vi "UsrProfiles-Parse param names.vi"(10 "key":string, 11 "Saved value":dbl) -> (3 "String":string)   [LabVIEW 2020]
uses:
  Typedefs/Movement mode.ctl
  Typedefs/Reference source.ctl
  Movement Correction/Typedefs/Control algorithm.ctl
  Typedefs/Channel Selector.ctl
  Typedefs/Line draw mode.ctl
  Typedefs/Imaging Protocols enum.ctl
  Typedefs/AOL modes.ctl
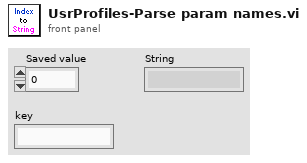
[diagram p1: front panel]
types:
  T1 = typedef "Movement mode.ctl" = enum16{"Move the frame", "Move the feature"}
  T2 = typedef "Reference source.ctl" = enum16{"Green channel", "Red channel"}
  T3 = typedef "Control algorithm.ctl" = enum16{"PID", "Kalman"}
  T4 = typedef "Channel Selector.ctl" = enum16{"Red Channel", "Green Channel", "Blended"}
  T5 = enum16{"Grayscale", "Binary", "Gradient", "Rainbow", "Temperature", "User Defined"}
  T6 = typedef "Line draw mode.ctl" = enum16{"Free draw", "Orthogonal"}
  T7 = typedef "Imaging Protocols enum.ctl" = enum16{"AOL Z-Stack", "Motor Z Stack", "Functional Acquisition", "Single Plane Acquisition", "Volume Acquisition", "Live Imaging", "Live Plane Imaging", "Live Volume Imaging"}
  T8 = typedef "AOL modes.ctl" = enum16{"Raster", "Structural", "Pointing", "Mini Scan", "Alignment"}
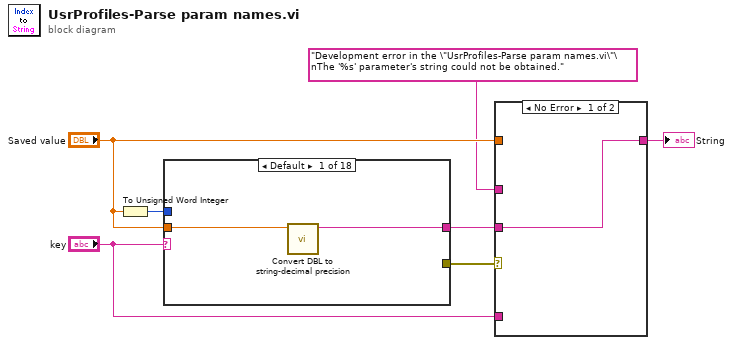
[diagram p0: block diagram]
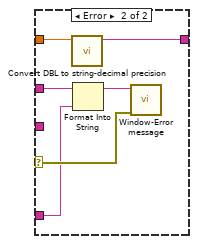
[diagram p2: hidden frame]
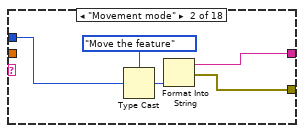
[diagram p3: hidden frame]
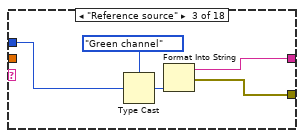
[diagram p4: hidden frame]
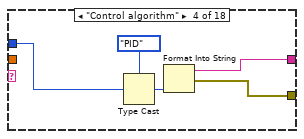
[diagram p5: hidden frame]
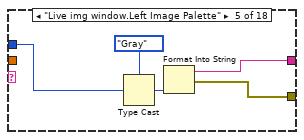
[diagram p6: hidden frame]
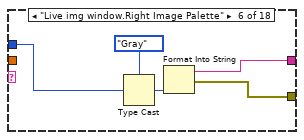
[diagram p7: hidden frame]
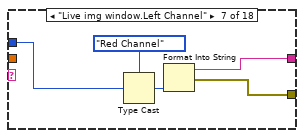
[diagram p8: hidden frame]
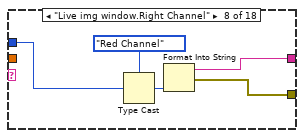
[diagram p9: hidden frame]
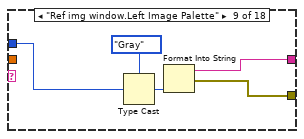
[diagram p10: hidden frame]
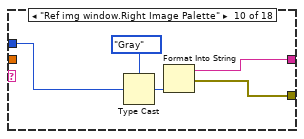
[diagram p11: hidden frame]
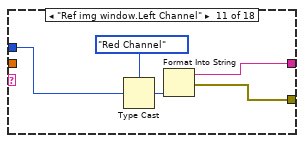
[diagram p12: hidden frame]
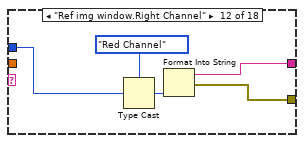
[diagram p13: hidden frame]
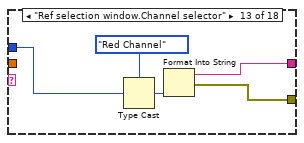
[diagram p14: hidden frame]
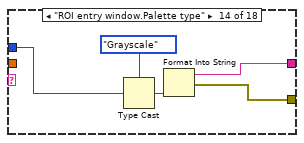
[diagram p15: hidden frame]
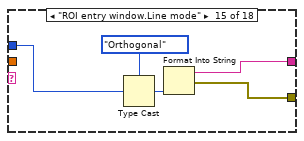
[diagram p16: hidden frame]
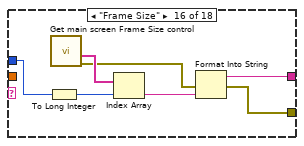
[diagram p17: hidden frame]
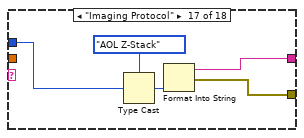
[diagram p18: hidden frame]
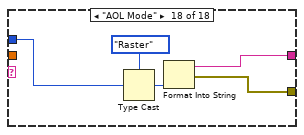
[diagram p19: hidden frame]
diagram:
  n1 = To Unsigned Word Integer(number="Saved value") -> (unsigned 16bit integer=w7:u16)
  n2 = case shown="Default" "key" {
    tunnel: w7 -> [_ w14 w19 w24 w29 w34 w39 w44 w49 w54 w59 w64 w69 w74 w79 w84 w91 w96]
    tunnel: [w8 w11 w17 w22 w27 w32 w37 w42 w47 w52 w57 w62 w67 w72 w77 w86 w89 w94] -> w4
    tunnel: [_ w10 w15 w20 w26 w31 w36 w41 w46 w51 w56 w61 w66 w71 w76 w85 w88 w93] -> w6
    tunnel: "Saved value" -> [w9 _ _ _ _ _ _ _ _ _ _ _ _ _ _ _ _ _]
    frame Default {
      n3 = call <userlib>:"Convert DBL to string-decimal precision.vi"("DBL Value"=w9) -> ("Converted to String"=w8:string)  [unwired: 10 in]
    }
    frame "Movement mode" {
      n4 = Type Cast(type=Movement_mode."Move the feature" ("Movement mode"), x=w14) -> (*(type *) &x=w13:T1)
      n5 = Format Into String(w13) -> (resulting string=w11:string, error out=w10:errorcluster)  [unwired: 3 in]
    }
    frame "Reference source" {
      n6 = Type Cast(type=Reference_source."Green channel" ("Reference Source"), x=w19) -> (*(type *) &x=w18:T2)
      n7 = Format Into String(w18) -> (resulting string=w17:string, error out=w15:errorcluster)  [unwired: 3 in]
    }
    frame "Control algorithm" {
      n8 = Type Cast(type=Control_algorithm."PID" ("Control algorithm"), x=w24) -> (*(type *) &x=w23:T3)
      n9 = Format Into String(w23) -> (resulting string=w22:string, error out=w20:errorcluster)  [unwired: 3 in]
    }
    frame "Live img window.Left Image Palette" {
      n10 = Type Cast(type=enum16{"Gray", "Red", "Green"}."Gray" ("Value"), x=w29) -> (*(type *) &x=w28:enum16{"Gray", "Red", "Green"})
      n11 = Format Into String(w28) -> (resulting string=w27:string, error out=w26:errorcluster)  [unwired: 3 in]
    }
    frame "Live img window.Right Image Palette" {
      n12 = Type Cast(type=enum16{"Gray", "Red", "Green"}."Gray" ("Value"), x=w34) -> (*(type *) &x=w33:enum16{"Gray", "Red", "Green"})
      n13 = Format Into String(w33) -> (resulting string=w32:string, error out=w31:errorcluster)  [unwired: 3 in]
    }
    frame "Live img window.Left Channel" {
      n14 = Type Cast(type=Channel_Selector."Red Channel" ("Value"), x=w39) -> (*(type *) &x=w38:T4)
      n15 = Format Into String(w38) -> (resulting string=w37:string, error out=w36:errorcluster)  [unwired: 3 in]
    }
    frame "Live img window.Right Channel" {
      n16 = Type Cast(type=Channel_Selector."Red Channel" ("Value"), x=w44) -> (*(type *) &x=w43:T4)
      n17 = Format Into String(w43) -> (resulting string=w42:string, error out=w41:errorcluster)  [unwired: 3 in]
    }
    frame "Ref img window.Left Image Palette" {
      n18 = Type Cast(type=enum16{"Gray", "Red", "Green"}."Gray" ("Value"), x=w49) -> (*(type *) &x=w48:enum16{"Gray", "Red", "Green"})
      n19 = Format Into String(w48) -> (resulting string=w47:string, error out=w46:errorcluster)  [unwired: 3 in]
    }
    frame "Ref img window.Right Image Palette" {
      n20 = Type Cast(type=enum16{"Gray", "Red", "Green"}."Gray" ("Value"), x=w54) -> (*(type *) &x=w53:enum16{"Gray", "Red", "Green"})
      n21 = Format Into String(w53) -> (resulting string=w52:string, error out=w51:errorcluster)  [unwired: 3 in]
    }
    frame "Ref img window.Left Channel" {
      n22 = Type Cast(type=Channel_Selector."Red Channel" ("Value"), x=w59) -> (*(type *) &x=w58:T4)
      n23 = Format Into String(w58) -> (resulting string=w57:string, error out=w56:errorcluster)  [unwired: 3 in]
    }
    frame "Ref img window.Right Channel" {
      n24 = Type Cast(type=Channel_Selector."Red Channel" ("Value"), x=w64) -> (*(type *) &x=w63:T4)
      n25 = Format Into String(w63) -> (resulting string=w62:string, error out=w61:errorcluster)  [unwired: 3 in]
    }
    frame "Ref selection window.Channel selector" {
      n26 = Type Cast(type=Channel_Selector."Red Channel" ("Value"), x=w69) -> (*(type *) &x=w68:T4)
      n27 = Format Into String(w68) -> (resulting string=w67:string, error out=w66:errorcluster)  [unwired: 3 in]
    }
    frame "ROI entry window.Palette type" {
      n28 = Type Cast(type=T5."Grayscale" ("Value"), x=w74) -> (*(type *) &x=w73:T5)
      n29 = Format Into String(w73) -> (resulting string=w72:string, error out=w71:errorcluster)  [unwired: 3 in]
    }
    frame "ROI entry window.Line mode" {
      n30 = Type Cast(type=Line_draw_mode."Orthogonal" ("Value"), x=w79) -> (*(type *) &x=w78:T6)
      n31 = Format Into String(w78) -> (resulting string=w77:string, error out=w76:errorcluster)  [unwired: 3 in]
    }
    frame "Frame Size" {
      n32 = To Long Integer(number=w84) -> (32bit integer=w83:i32)
      n33 = call "Get main screen Frame Size control.vi"() -> ("error out"=w80:errorcluster, "Strings []"=w81:string[])  [unwired: 9 in, 1 out]
      n34 = Index Array(array=w81, index=w83) -> (element=w82:string)
      n35 = Format Into String(error in=w80, w82) -> (resulting string=w86:string, error out=w85:errorcluster)  [unwired: 2 in]
    }
    frame "Imaging Protocol" {
      n36 = Type Cast(type=Imaging_Protocols_enum."AOL Z-Stack" ("Imaging Protocol"), x=w91) -> (*(type *) &x=w90:T7)
      n37 = Format Into String(w90) -> (resulting string=w89:string, error out=w88:errorcluster)  [unwired: 3 in]
    }
    frame "AOL Mode" {
      n38 = Type Cast(type=AOL_modes."Raster" ("AOL Mode"), x=w96) -> (*(type *) &x=w95:T8)
      n39 = Format Into String(w95) -> (resulting string=w94:string, error out=w93:errorcluster)  [unwired: 3 in]
    }
  }
  n40 = case shown="No Error" w6 {
    selector: w6 -> [_ w99]
    tunnel: "Saved value" -> [_ w103]
    tunnel: w4 -> [w97 _]
    tunnel: [w97 w102] -> w3
    tunnel: "Development error in the \"UsrProfiles-Parse param names.vi\"\nThe '%s' parameter's string could not be obtained." ("Message") -> [_ w101]
    tunnel: "key" -> [_ w98]
    frame No Error {
    }
    frame Error {
      n41 = call <userlib>:"Convert DBL to string-decimal precision.vi"("DBL Value"=w103) -> ("Converted to String"=w102:string)  [unwired: 10 in]
      n42 = Format Into String(initial string=w101, w98) -> (resulting string=w100:string)  [unwired: 2 in, 1 out]
      n43 = call "Window-Error message.vi"("error in (no error)"=w99, "Message"=w100) -> ()  [unwired: 9 in, 1 out]
    }
  }
  "String" <- w3
